vi "Superimpose Crosshairs.vi"(1 "Grid Line Color":u32(colorbox)=16711680, 2 "Refnum in":T1) -> (0 "Refnum out":T1(plugin-control))   [LabVIEW 2011]
uses:
  <vilib>/vision/Image Controls.llb/IMAQ Image.ctl
panel:
  out "error out":errorcluster
  in  "error in":errorcluster
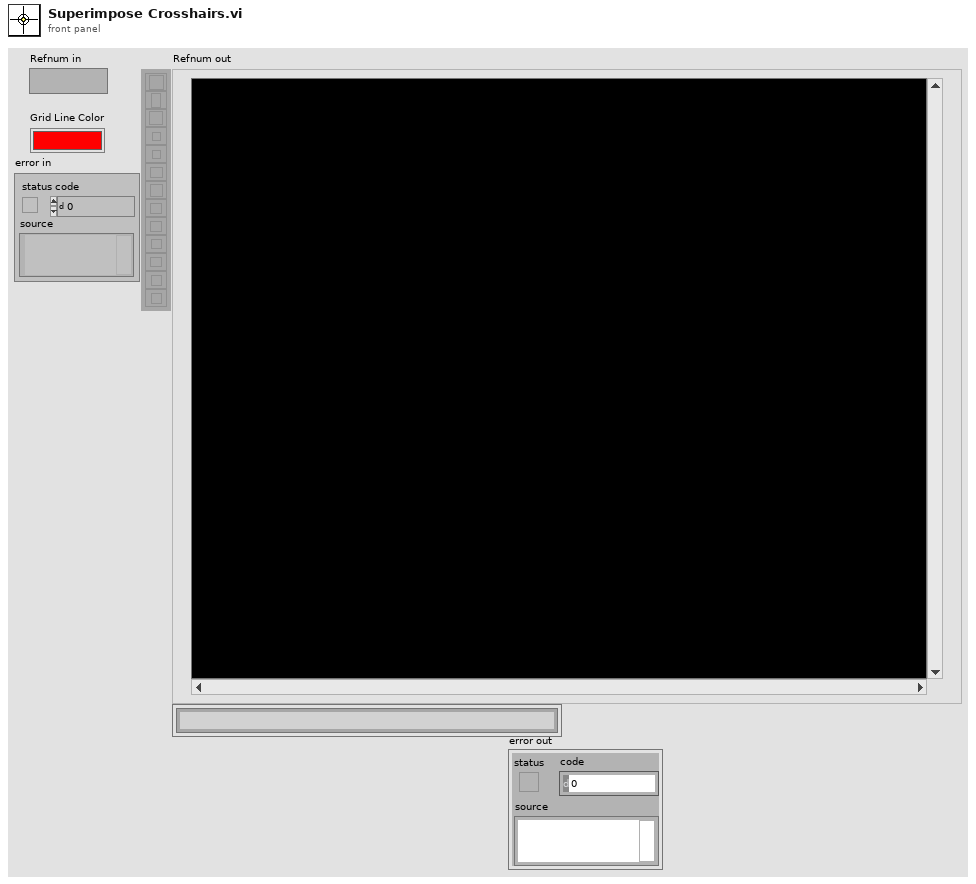
[diagram p1: front panel]
types:
  T1 = typedef "IMAQ Image.ctl" = refnum<image>
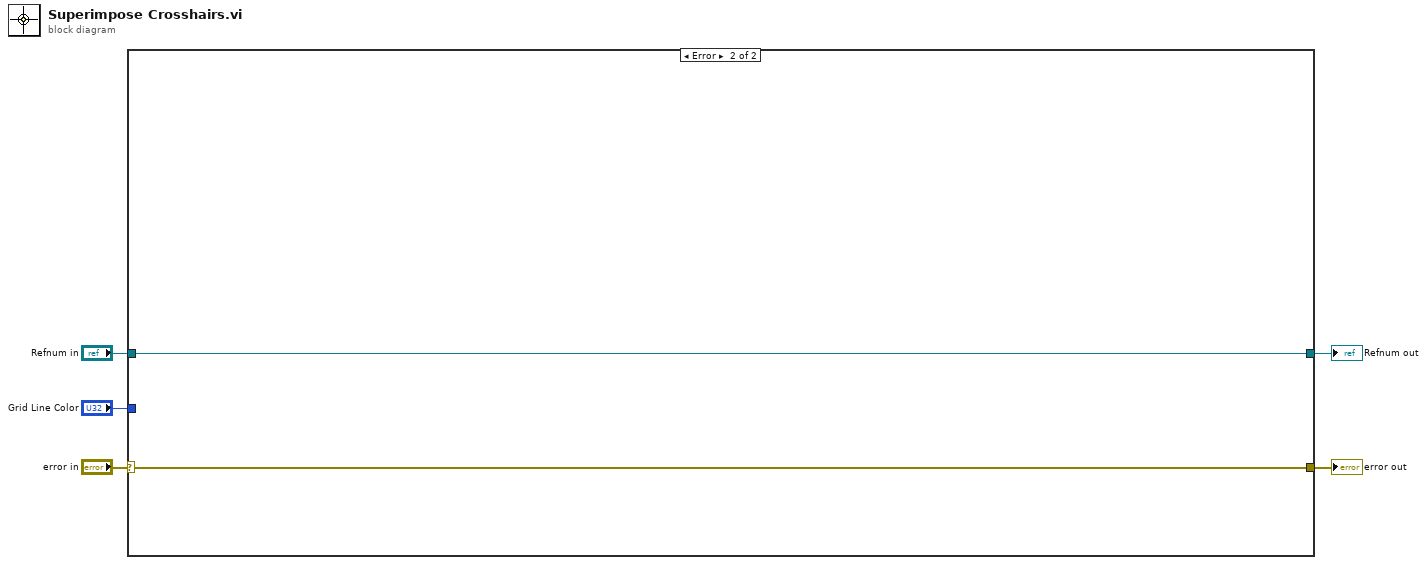
[diagram p0: block diagram]
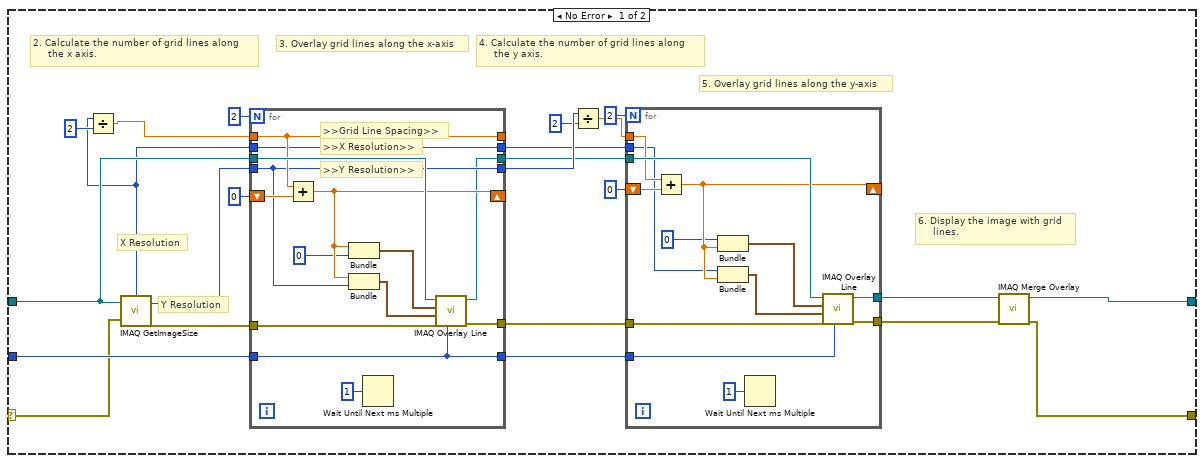
[diagram p2: hidden frame]
diagram:
  n1 = case shown="Error" "error in" {
    selector: "error in" -> [w8 w57]
    tunnel: "Refnum in" -> [w28 w56]
    tunnel: "Grid Line Color" -> [w16 _]
    tunnel: [w7 w56] -> w2
    tunnel: [w6 w57] -> w1
    frame No Error {
      # "X Resolution"
      # "Y Resolution"
      # "6. Display the image with grid\n     lines."
      # "5. Overlay grid lines along the y-axis"
      # "4. Calculate the number of grid lines along\n     the y axis."
      # "3. Overlay grid lines along the x-axis"
      # "2. Calculate the number of grid lines along\n     the x axis."
      n2 = call "IMAQ GetImageSize"("Image"=w28, "error in (no error)"=w8) -> ("Y Resolution"=w12:i32, "X Resolution"=w23:i32, "error out"=w9:errorcluster)  [unwired: 2 in]
      n3 = Divide(x=w23, y=2) -> (x/y=w22:dbl)
      n4 = for {
        N: 2 -> [_]
        tunnel: w9 -> [w55]
        tunnel: [w54] -> w10
        tunnel: w28 -> [w53]
        tunnel: [w42] -> w11
        tunnel: w22 -> [w52]
        tunnel: [w52] -> _
        tunnel: [w48] -> w26
        tunnel: w12 -> [w48]
        shift-right: [w50] -> _
        shift-left: 0 -> [w51]
        tunnel: [w45] -> w15
        tunnel: w23 -> [w45]
        tunnel: w16 -> [w44]
        tunnel: [w44] -> w17
        # ">>Y Resolution>>"
        # ">>X Resolution>>"
        # ">>Grid Line Spacing>>"
        n5 = Add(x=w52, y=w51) -> (x+y=w50:dbl)
        n6 = Bundle(w50, 0) -> (w47:cluster{dbl, i32})  [unwired: 1 in]
        n7 = Bundle(w50, "Y Resolution"=w48) -> (w46:cluster{dbl, "Y Resolution":i32})  [unwired: 1 in]
        n8 = Wait Until Next ms Multiple(millisecond multiple=u32 1) -> ()  [unwired: 1 out]
        n9 = call "IMAQ Overlay Line"("Color"=w44, "error in (no error)"=w55, "End Point"=w46, "Start Point"=w47, "Image"=w53) -> ("error out"=w54:errorcluster, "Image Out"=w42:T1)  [unwired: 5 in]
      }
      n10 = Divide(x=w26, y=2) -> (x/y=w27:dbl)
      n11 = for {
        N: 2 -> [_]
        tunnel: w10 -> [w41]
        tunnel: [w40] -> w19
        tunnel: w11 -> [w39]
        shift-right: [w36] -> _
        shift-left: 0 -> [w38]
        tunnel: w27 -> [w37]
        tunnel: w15 -> [w34]
        tunnel: [w31] -> w18
        tunnel: w17 -> [w30]
        n12 = Add(x=w37, y=w38) -> (x+y=w36:dbl)
        n13 = Bundle(0, w36) -> (w33:cluster{i32, dbl})  [unwired: 1 in]
        n14 = Bundle("X Resolution"=w34, w36) -> (w32:cluster{"X Resolution":i32, dbl})  [unwired: 1 in]
        n15 = Wait Until Next ms Multiple(millisecond multiple=u32 1) -> ()  [unwired: 1 out]
        n16 = call "IMAQ Overlay Line"("Color"=w30, "error in (no error)"=w41, "End Point"=w32, "Start Point"=w33, "Image"=w39) -> ("error out"=w40:errorcluster, "Image Out"=w31:T1)  [unwired: 5 in]
      }
      n17 = call "IMAQ Merge Overlay"("error in (no error)"=w19, "Image Src"=w18) -> ("error out"=w6:errorcluster, "Image Dst Out"=w7:T1)  [unwired: 8 in]
    }
    frame Error {
    }
  }
  "Refnum out" <- w2
  "error out" <- w1
